vi "Test.vi"() -> ()   [LabVIEW 2015, in "ReDeX.lvlib"]
uses:
  ReDeX.lvlib
  subvi/SensorInfo.ctl
panel:
  out "Temperature":dbl format="%#_3f °C"
  out "Current":dbl format="%#_3p A"
  out "Voltage":dbl format="%#_3p V"
  out "Nodes":cluster{"ID":string, "Type":string}[](array[cluster])
  out "Hub Temperature":dbl format="%#_g °C"
  in  "Pause":bool
  out "Status":u32(ring)=1 items=["MeasurementStarted", "MeasurementStopped", "MeasurementError"]
  out "Error Message":string
  out "Voltammogram 1":T1(graph)
  out "Testpoints":T3(array[cluster])
  out "Temperature":dbl format="%#_3p °C"
  out "pH Value":dbl format="%#_4p"
  out "ORP Value":dbl format="%#_4p V"
  out "Admittance":dbl format="%#_4p S"
  out "Current":dbl format="%#_4p A"
  out "Voltage":dbl format="%#_4p V"
  in  "Stop":bool
  in  "Host":string="redex-hub.local"
  # "Node Status"
  # "Testpoint 1"
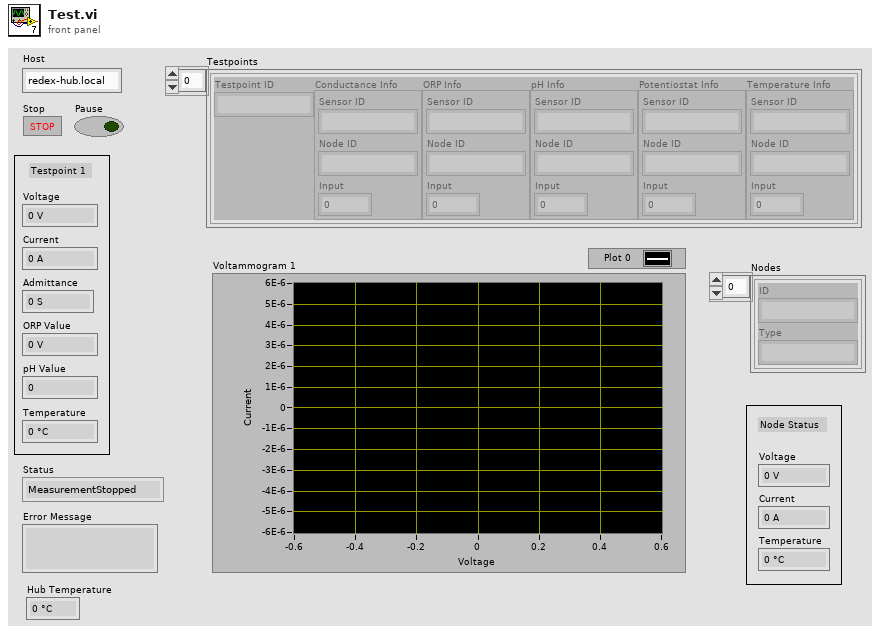
[diagram p1: front panel]
types:
  T1 = cluster{"Raw Voltage":dbl[], "Raw Current":dbl[]}
  T2 = typedef "ReDeX.lvlib/SensorInfo.ctl" = cluster{"Sensor ID":string, "Node ID":string, "Input":u32}
  T3 = cluster{"Testpoint ID":string, "Conductance Info":T2, "ORP Info":T2, "pH Info":T2, "Potentiostat Info":T2, "Temperature Info":T2}[]
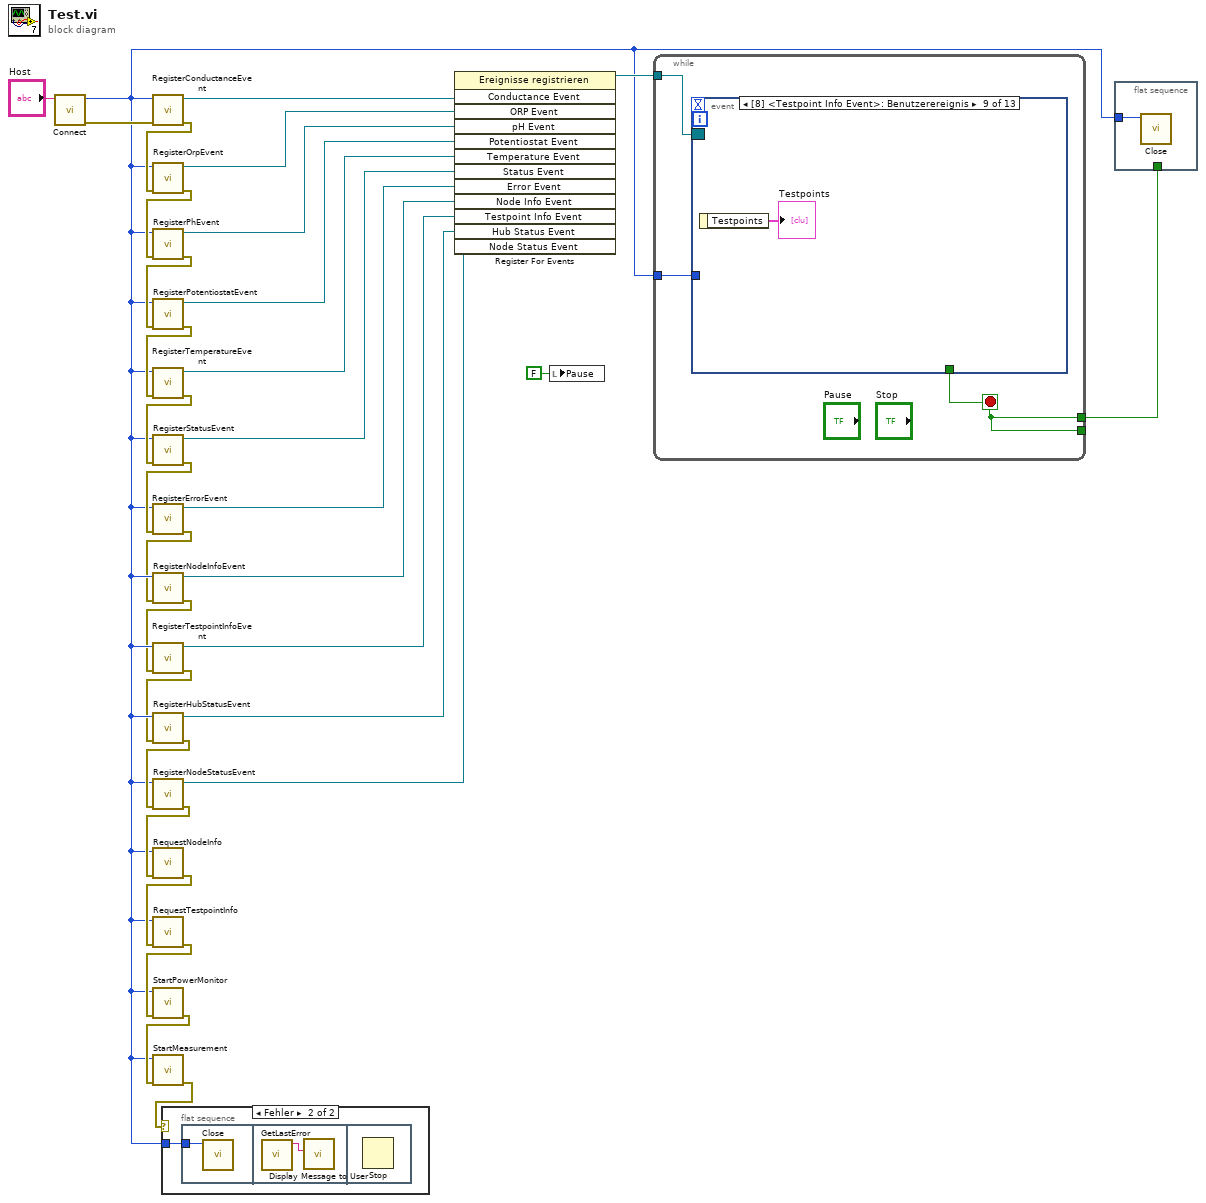
[diagram p0: block diagram]
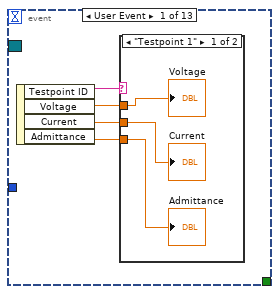
[diagram p3: hidden frame]
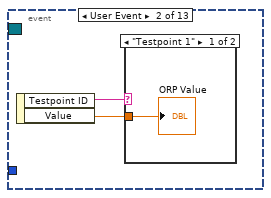
[diagram p5: hidden frame]
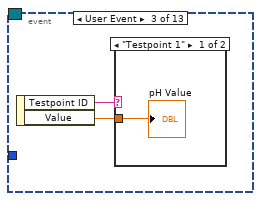
[diagram p7: hidden frame]
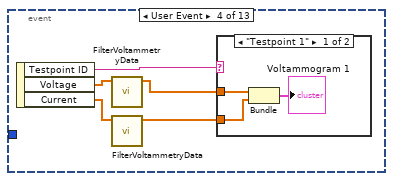
[diagram p9: hidden frame]
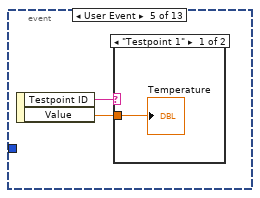
[diagram p11: hidden frame]
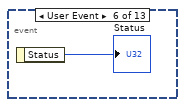
[diagram p13: hidden frame]
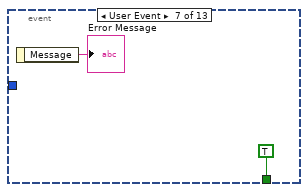
[diagram p14: hidden frame]
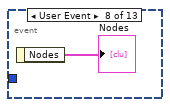
[diagram p15: hidden frame]
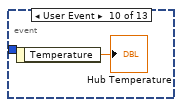
[diagram p16: hidden frame]
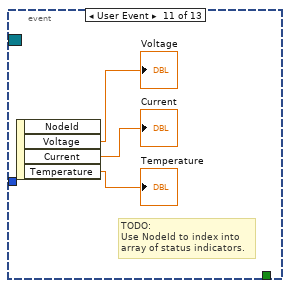
[diagram p17: hidden frame]
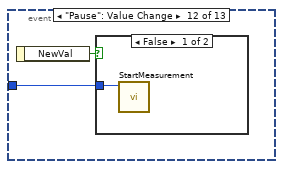
[diagram p18: hidden frame]
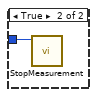
[diagram p19: hidden frame]
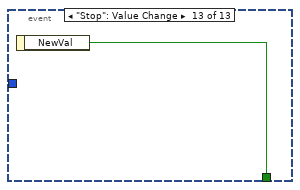
[diagram p20: hidden frame]
diagram:
  n1 = call "Connect.vi"("host"="Host") -> ("error out"=w29:errorcluster, "handle"=w6:u64)  [unwired: 9 in]
  n2 = call "RegisterConductanceEvent.vi"("error in (no error)"=w29, "handle"=w6) -> ("error out"=w28:errorcluster, "Conductance Event"=w30:refnum<user-event>)  [unwired: 8 in]
  n3 = call "RegisterOrpEvent.vi"("error in (no error)"=w28, "handle"=w6) -> ("error out"=w26:errorcluster, "ORP Event"=w27:refnum<user-event>)  [unwired: 8 in]
  n4 = call "RegisterPhEvent.vi"("error in (no error)"=w26, "handle"=w6) -> ("error out"=w21:errorcluster, "pH Event"=w25:refnum<user-event>)  [unwired: 8 in]
  n5 = call "RegisterPotentiostatEvent.vi"("error in (no error)"=w21, "handle"=w6) -> ("error out"=w22:errorcluster, "Potentiostat Event"=w24:refnum<user-event>)  [unwired: 8 in]
  n6 = call "RegisterTemperatureEvent.vi"("error in (no error)"=w22, "handle"=w6) -> ("error out"=w20:errorcluster, "Temperature Event"=w23:refnum<user-event>)  [unwired: 8 in]
  n7 = call "RegisterStatusEvent.vi"("error in (no error)"=w20, "handle"=w6) -> ("error out"=w19:errorcluster, "Status Event"=w17:refnum<user-event>)  [unwired: 8 in]
  n8 = call "RegisterErrorEvent.vi"("error in (no error)"=w19, "handle"=w6) -> ("error out"=w5:errorcluster, "Error Event"=w18:refnum<user-event>)  [unwired: 8 in]
  n9 = call "RegisterNodeInfoEvent.vi"("error in (no error)"=w5, "handle"=w6) -> ("error out"=w1:errorcluster, "Node Info Event"=w3:refnum<user-event>)  [unwired: 8 in]
  n10 = call "RegisterTestpointInfoEvent.vi"("error in (no error)"=w1, "handle"=w6) -> ("error out"=w4:errorcluster, "Testpoint Info Event"=w2:refnum<user-event>)  [unwired: 8 in]
  n11 = call "RegisterHubStatusEvent.vi"("error in (no error)"=w4, "handle"=w6) -> ("error out"=w11:errorcluster, "Hub Status Event"=w9:refnum<user-event>)  [unwired: 8 in]
  n12 = call "RegisterNodeStatusEvent.vi"("error in (no error)"=w11, "handle"=w6) -> ("error out"=w8:errorcluster, "Node Status Event"=w10:refnum<user-event>)  [unwired: 8 in]
  n13 = call "RequestNodeInfo.vi"("error in (no error)"=w8, "handle"=w6) -> ("error out"=w7:errorcluster)  [unwired: 9 in]
  n14 = call "RequestTestpointInfo.vi"("error in (no error)"=w7, "handle"=w6) -> ("error out"=w13:errorcluster)  [unwired: 9 in]
  n15 = call "StartPowerMonitor.vi"("error in (no error)"=w13, "handle"=w6) -> ("error out"=w12:errorcluster)  [unwired: 9 in]
  n16 = call "StartMeasurement.vi"("error in (no error)"=w12, "handle"=w6) -> ("error out"=w15:errorcluster)  [unwired: 9 in]
  n17 = case shown="Fehler" w15 {
    tunnel: w6 -> [_ w33]
    frame No Error {
    }
    frame Error {
      n18 = flat-sequence {
        tunnel: w33 -> [w34]
        frame #0 {
          n19 = call "Close.vi"("handle"=w34) -> ()  [unwired: 10 in, 1 out]
        }
        frame #1 {
          n20 = call "GetLastError.vi"() -> ("function return"=w35:string)  [unwired: 10 in, 1 out]
          n21 = call "Display Message to User"("Message"=w35) -> ()  [unwired: 9 in, 2 out]
        }
        frame #2 {
          n22 = Stop() -> ()  [unwired: 1 in]
        }
      }
    }
  }
  n23 = register-events(w30, w27, w25, w24, w23, w17, w18, w3, w2, w9, w10) -> (reference out=w31:refnum<event-registration>)  [unwired: 2 in, 1 out]
  n24 = local write "Pause"(FALSE ("Pause")) -> ()
  n25 = while {
    tunnel: w31 -> [w38]
    tunnel: [w36] -> w16
    tunnel: [w36] -> _
    tunnel: w6 -> [w37]
    stop <- w36 stop-if-true
    n26 = event shown="[8] <Testpoint Info Event>: Benutzerereignis" {
      selector: w38 -> [_ _ _ _ _ _ _ _ _ _ _ _ _]
      dyn-events: _ -> [_ _ _ _ _ _ _ _ _ _ _ _ _]
      timeout: _ -> [_ _ _ _ _ _ _ _ _ _ _ _ _]
      tunnel: [_ _ _ _ _ _ TRUE _ _ _ _ _ w76] -> w36
      tunnel: w37 -> [_ _ _ _ _ _ _ _ _ _ _ w72 _]
      event User Event {
        n27 = event-data() -> ("Testpoint ID"=w42:string, "Voltage"=w41:dbl, "Current"=w40:dbl, "Admittance"=w39:dbl)  [unwired: 1 in]
        n28 = case shown="\"Testpoint 1\"" w42 {
          tunnel: w41 -> [w45 _]
          tunnel: w40 -> [w44 _]
          tunnel: w39 -> [w43 _]
          frame "Testpoint 1" {
            "Voltage" <- w45
            "Current" <- w44
            "Admittance" <- w43
          }
          frame Default {
          }
        }
      }
      event User Event {
        n29 = event-data() -> ("Testpoint ID"=w47:string, "Value"=w46:dbl)  [unwired: 1 in]
        n30 = case shown="\"Testpoint 1\"" w47 {
          tunnel: w46 -> [w48 _]
          frame "Testpoint 1" {
            "ORP Value" <- w48
          }
          frame Default {
          }
        }
      }
      event User Event {
        n31 = event-data() -> ("Testpoint ID"=w50:string, "Value"=w49:dbl)  [unwired: 1 in]
        n32 = case shown="\"Testpoint 1\"" w50 {
          tunnel: w49 -> [w51 _]
          frame "Testpoint 1" {
            "pH Value" <- w51
          }
          frame Default {
          }
        }
      }
      event User Event {
        n33 = event-data() -> ("Testpoint ID"=w56:string, "Voltage"=w55:dbl[], "Current"=w54:dbl[])  [unwired: 1 in]
        n34 = call "FilterVoltammetryData.vi"("Input"=w55) -> ("Output"=w53:dbl[])  [unwired: 9 in, 1 out]
        n35 = call "FilterVoltammetryData.vi"("Input"=w54) -> ("Output"=w52:dbl[])  [unwired: 9 in, 1 out]
        n36 = case shown="\"Testpoint 1\"" w56 {
          tunnel: w53 -> [w58 _]
          tunnel: w52 -> [w57 _]
          frame "Testpoint 1" {
            n37 = Bundle("Output"=w58, "Output"=w57) -> (→"Voltammogram 1":cluster{"Output":dbl[], "Output":dbl[]})  [unwired: 1 in]
          }
          frame Default {
          }
        }
      }
      event User Event {
        n38 = event-data() -> ("Testpoint ID"=w60:string, "Value"=w61:dbl)  [unwired: 1 in]
        n39 = case shown="\"Testpoint 1\"" w60 {
          tunnel: w61 -> [w62 _]
          frame "Testpoint 1" {
            "Temperature" <- w62
          }
          frame Default {
          }
        }
      }
      event User Event {
        n40 = event-data() -> ("Status"=→"Status":i32)  [unwired: 1 in]
      }
      event User Event {
        n41 = event-data() -> ("Message"=→"Error Message":string)  [unwired: 1 in]
      }
      event User Event {
        n42 = event-data() -> ("Nodes"=→"Nodes":cluster{"ID":string, "Type":string}[])  [unwired: 1 in]
      }
      event User Event {
        n43 = event-data() -> ("Testpoints"=→"Testpoints":T3)  [unwired: 1 in]
      }
      event User Event {
        n44 = event-data() -> ("Temperature"=→"Hub Temperature":dbl)  [unwired: 1 in]
      }
      event User Event {
        # "TODO:\nUse NodeId to index into\narray of status indicators."
        n45 = event-data() -> ("Voltage"=→"Voltage":dbl, "Current"=→"Current":dbl, "Temperature"=→"Temperature":dbl)  [unwired: 1 in, 1 out]
      }
      event "Pause": Value Change {
        n46 = event-data() -> ("NewVal"=w73:bool)  [unwired: 1 in]
        n47 = case shown="False" w73 {
          tunnel: w72 -> [w74 w75]
          frame False {
            n48 = call "StartMeasurement.vi"("handle"=w74) -> ()  [unwired: 10 in, 1 out]
          }
          frame True {
            n49 = call "StopMeasurement.vi"("handle"=w75) -> ()  [unwired: 10 in, 1 out]
          }
        }
      }
      event "Stop": Value Change {
        n50 = event-data() -> ("NewVal"=w76:bool)  [unwired: 1 in]
      }
    }
  }
  n51 = flat-sequence {
    tunnel: w6 -> [w77]
    tunnel: w16 -> [_]
    frame #0 {
      n52 = call "Close.vi"("handle"=w77) -> ()  [unwired: 10 in, 1 out]
    }
  }
